vi "xijk_hide_template_boxes.vi"(9 "number":u8, 10 "template selector in":u16, 11 "spectra parameters in":T2={"Booleans"={"Notch filtering"=FALSE, "Unknown detector"=FALSE, "Dual band filters"=FALSE, "Dual emission by cubes"=FALSE, "FRET"=FALSE}, "Integers"={"Light source"=0, "Number of fluorophores"=0, "Wavelength of laser (nm) 1"=0, "Broadness of laser (nm) 1"=0.0, "Wavelength of laser (nm) 2"=0, "Broadness of laser (nm) 2"=0.0, "Template"=1}, "Doubles"={"Molar extinction 1"=1.0, "Molar extinction 2"=1.0, "Quantum efficiency 1"=1.0, "Quantum efficiency 2"=1.0}}) -> (0 "table for calculation automagic out":i32[](array[numeric]), 1 "enable array out":T1(array[ring]), 2 "concatenated string":string, 3 "spectra parameters out":T2={"Booleans"={"Notch filtering"=FALSE, "Unknown detector"=FALSE, "Dual band filters"=FALSE, "Dual emission by cubes"=FALSE, "FRET"=FALSE}, "Integers"={"Light source"=0, "Number of fluorophores"=0, "Wavelength of laser (nm) 1"=0, "Broadness of laser (nm) 1"=0.0, "Wavelength of laser (nm) 2"=0, "Broadness of laser (nm) 2"=0.0, "Template"=1}, "Doubles"={"Molar extinction 1"=1.0, "Molar extinction 2"=1.0, "Quantum efficiency 1"=1.0, "Quantum efficiency 2"=1.0}})   [LabVIEW 2010]
uses:
  Type Def/spectra_parameters.ctl
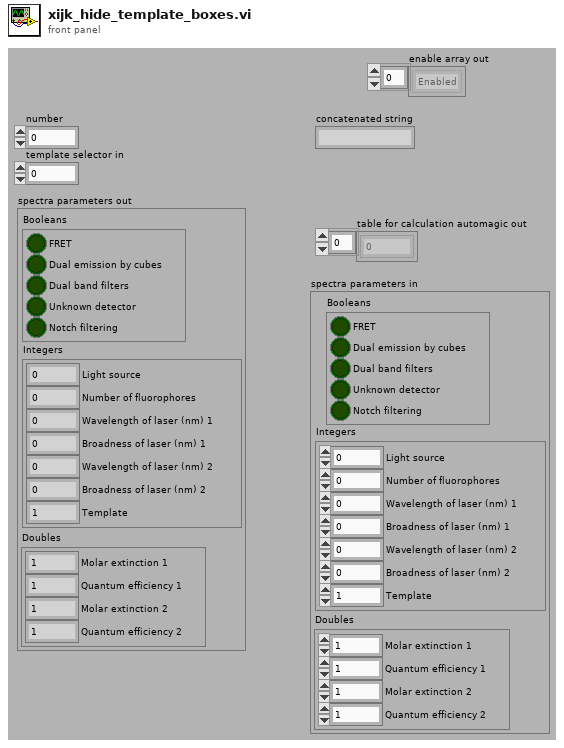
[diagram p1: front panel]
types:
  T1 = enum8{"Enabled", "Disabled", "Disabled and Grayed Out"}[]
  T2 = typedef "spectra_parameters.ctl" = cluster{"Booleans":cluster{"Notch filtering":bool, "Unknown detector":bool, "Dual band filters":bool, "Dual emission by cubes":bool, "FRET":bool}, "Integers":cluster{"Light source":u16, "Number of fluorophores":u16, "Wavelength of laser (nm) 1":u16, "Broadness of laser (nm) 1":sgl, "Wavelength of laser (nm) 2":u16, "Broadness of laser (nm) 2":sgl, "Template":u16}, "Doubles":cluster{"Molar extinction 1":sgl, "Molar extinction 2":sgl, "Quantum efficiency 1":sgl, "Quantum efficiency 2":sgl}}
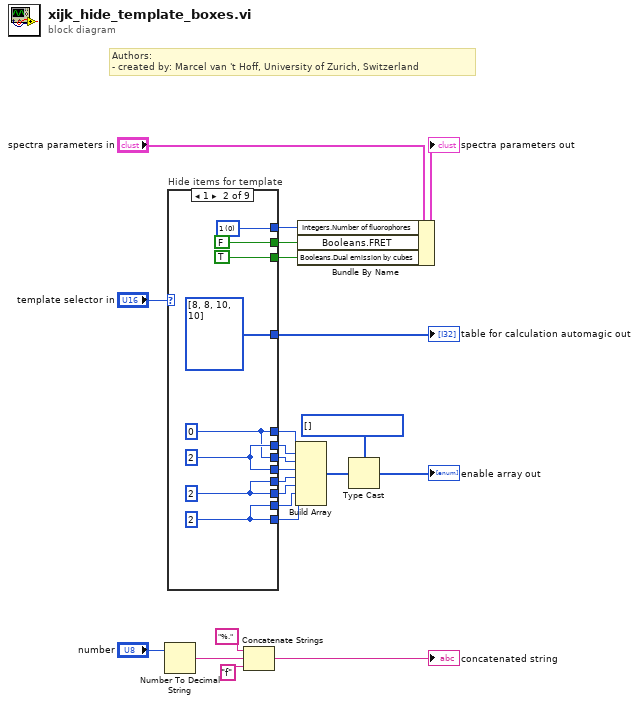
[diagram p0: block diagram]
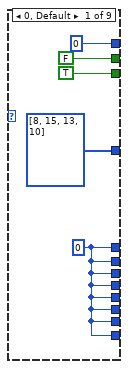
[diagram p2: hidden frame]
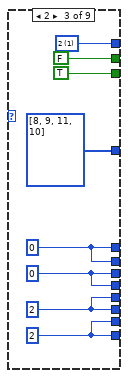
[diagram p3: hidden frame]
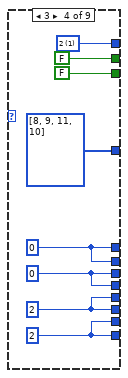
[diagram p4: hidden frame]
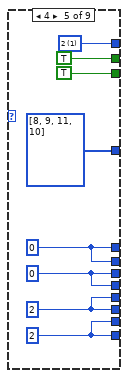
[diagram p5: hidden frame]
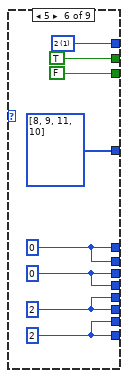
[diagram p6: hidden frame]
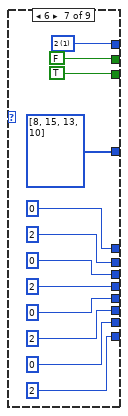
[diagram p7: hidden frame]
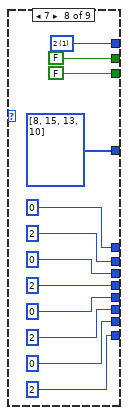
[diagram p8: hidden frame]
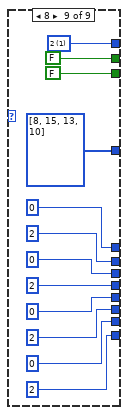
[diagram p9: hidden frame]
diagram:
  w2 = T1 [] items=["Enabled", "Disabled", "Disabled and Grayed Out"]
  # "Authors: \n- created by: Marcel van 't Hoff, University of Zurich, Switzerland"
  n1 = Number To Decimal String(number="number") -> (decimal integer string=w22:string)  [unwired: 1 out]
  n2 = case "Hide items for template" shown="1" "template selector in" {
    tunnel: [w28 w29 w44 w52 w60 w68 u8 0 ("Désactivé") u8 0 ("Désactivé") u8 0 ("Désactivé")] -> w17
    tunnel: [w28 w30 w44 w52 w60 w68 u8 2 ("Désactivé") u8 2 ("Désactivé") u8 2 ("Désactivé")] -> w16
    tunnel: [w28 w29 w43 w51 w59 w67 u8 0 ("Désactivé") u8 0 ("Désactivé") u8 0 ("Désactivé")] -> w15
    tunnel: [w28 w30 w43 w51 w59 w67 u8 2 ("Désactivé") u8 2 ("Désactivé") u8 2 ("Désactivé")] -> w14
    tunnel: [w28 w36 w42 w50 w58 w66 u8 0 ("Désactivé") u8 0 ("Désactivé") u8 0 ("Désactivé")] -> w13
    tunnel: [w28 w36 w42 w50 w58 w66 u8 2 ("Désactivé") u8 2 ("Désactivé") u8 2 ("Désactivé")] -> w12
    tunnel: [w28 w35 w41 w49 w57 w65 u8 0 ("Désactivé") u8 0 ("Désactivé") u8 0 ("Désactivé")] -> w11
    tunnel: [w28 w35 w41 w49 w57 w65 u8 2 ("Désactivé") u8 2 ("Désactivé") u8 2 ("Désactivé")] -> w10
    tunnel: [i32[] [8, 15, 13, 10] i32[] [8, 8, 10, 10] i32[] [8, 9, 11, 10] i32[] [8, 9, 11, 10] i32[] [8, 9, 11, 10] i32[] [8, 9, 11, 10] i32[] [8, 15, 13, 10] i32[] [8, 15, 13, 10] i32[] [8, 15, 13, 10]] -> w9
    tunnel: [u16 0 ("Number of fluorophores") w33 w39 w47 w55 w63 w71 w83 w95] -> w8
    tunnel: [FALSE ("FRET") FALSE ("FRET") FALSE ("FRET") FALSE ("FRET") TRUE ("FRET") TRUE ("FRET") FALSE ("FRET") FALSE ("FRET") FALSE ("FRET")] -> w7
    tunnel: [TRUE ("FRET") TRUE ("FRET") TRUE ("FRET") FALSE ("FRET") TRUE ("FRET") FALSE ("FRET") TRUE ("FRET") FALSE ("FRET") FALSE ("FRET")] -> w6
    frame 0, Default {
      w28 = u8 0 ("Désactivé")
    }
    frame 1 {
      w33 = u16 0 items=["1", "2"] ("Number of fluorophores")
      w35 = u8 2 ("Désactivé")
      w30 = u8 2 ("Désactivé")
      w36 = u8 2 ("Désactivé")
      w29 = u8 0 ("Désactivé")
    }
    frame 2 {
      w39 = u16 1 items=["1", "2"] ("Number of fluorophores")
      w41 = u8 2 ("Désactivé")
      w43 = u8 0 ("Désactivé")
      w42 = u8 2 ("Désactivé")
      w44 = u8 0 ("Désactivé")
    }
    frame 3 {
      w47 = u16 1 items=["1", "2"] ("Number of fluorophores")
      w49 = u8 2 ("Désactivé")
      w51 = u8 0 ("Désactivé")
      w50 = u8 2 ("Désactivé")
      w52 = u8 0 ("Désactivé")
    }
    frame 4 {
      w55 = u16 1 items=["1", "2"] ("Number of fluorophores")
      w57 = u8 2 ("Désactivé")
      w59 = u8 0 ("Désactivé")
      w58 = u8 2 ("Désactivé")
      w60 = u8 0 ("Désactivé")
    }
    frame 5 {
      w63 = u16 1 items=["1", "2"] ("Number of fluorophores")
      w65 = u8 2 ("Désactivé")
      w67 = u8 0 ("Désactivé")
      w66 = u8 2 ("Désactivé")
      w68 = u8 0 ("Désactivé")
    }
    frame 6 {
      w71 = u16 1 items=["1", "2"] ("Number of fluorophores")
    }
    frame 7 {
      w83 = u16 1 items=["1", "2"] ("Number of fluorophores")
    }
    frame 8 {
      w95 = u16 1 items=["1", "2"] ("Number of fluorophores")
    }
  }
  "table for calculation automagic out" <- w9
  n3 = Concatenate Strings("%." ("chaîne"), w22, "f" ("chaîne")) -> (→"concatenated string":string)
  n4 = Build Array(w17, w16, w15, w14, w13, w12, w11, w10) -> (w3:u8[])
  n5 = Bundle By Name(cluster="spectra parameters in", "Integers.Number of fluorophores"=w8, "Booleans.FRET"=w7, "Booleans.Dual emission by cubes"=w6) -> (→"spectra parameters out":T2)
  n6 = Type Cast(type=w2, x=w3) -> (*(type *) &x=→"enable array out":T1)
